vi "GenerateCode.vi"(1 "Terms":T1[](array[typedef]), 3 "Diagram":refnum<vi>, 5 "XRef":refnum<vi>, 6 "State In":T4={"Input Type"=variant(dbl 0.0), "Selection"=0, "Element Names"=[], "Type Strings"=[], "Element Types"=[]}) -> (0 "Generated Code?":bool, 2 "State Out":T4={"Input Type"=variant(dbl 0.0), "Selection"=0, "Element Names"=[], "Type Strings"=[], "Element Types"=[]}, 4 "Reply":string[](array[string]))   [LabVIEW 2015, in "Construct-Tagged-Union.xnode"]
doc: "This ability VI is called when it is time to define the execution behavior of your XNode via LabVIEW's scripting API. This VI is only called when you have previously informed LabVIEW that you need to script through a GenerateCode reply. Diagram is a reference to a diagram of a temporary VI. This diagram contains exactly one front panel terminal for each terminal of your XNode. Terms is an array of pairs of Term IDs and terminal references. LabVIEW will copy code scripted into this diagram into your XNode and connect everything to the correct terminals. The front panel terminals that are on this diagram are special in that they can only be on the top level diagram.\n \n Generate Code? is used to tell LabVIEW whether or not you want to copy the scripted diagram over. If there is an error and you wish not to commit the changes, then the old XNode behavior will be left unchanged. If you set Generate Code? to false, then this VI will be called again next time type propagation is run. Otherwise, it will not be called until you indicate that it should be through the reply on another ability VI.\n \n Because the diagram you are scripting into is separate from the VI containing the XNode instance, type propagation and the data manager will run on the temporary VI after each scripting call.\n \n You should not use the Copy scripting method to move code into the temporary VI. This will adversely affect the user's clipboard. You should use the Move scripting method instead.\n\nDefault behavior: None.\n\nThis ability does not provide UI and OS messages are not handled.\n\nSee also: ModifyCode"
uses:
  Construct-Tagged-Union.xnode
  State.ctl
  <vilib>/XNodeSupport/XNodeTermIDPair.ctl
  <vilib>/XNodeSupport/XNodeTermRef.ctl
  <vilib>/XNodeSupport/XNodeString.ctl
  <vilib>/Erdos Miller/LV-Scripting/LV-Scripting.lvlib
  <vilib>/XNodeSupport/NI_XNodeSupport.lvlib
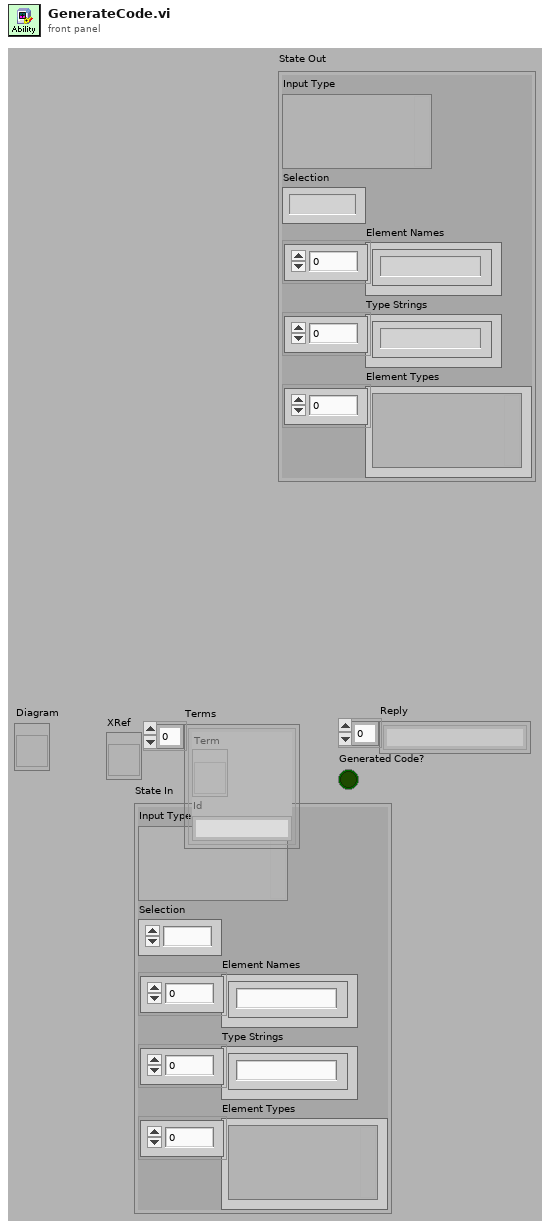
[diagram p1: front panel]
types:
  T1 = typedef "NI_XNodeSupport.lvlib/XNodeTermIDPair.ctl" = cluster{"Term":T2, "Id":T3}
  T2 = typedef "NI_XNodeSupport.lvlib/XNodeTermRef.ctl" = refnum<vi>
  T3 = typedef "NI_XNodeSupport.lvlib/XNodeString.ctl" = string
  T4 = typedef "Construct-Tagged-Union.xnode/State.ctl" = cluster{"Input Type":variant, "Selection":i32, "Element Names":string[], "Type Strings":string[], "Element Types":variant[]}
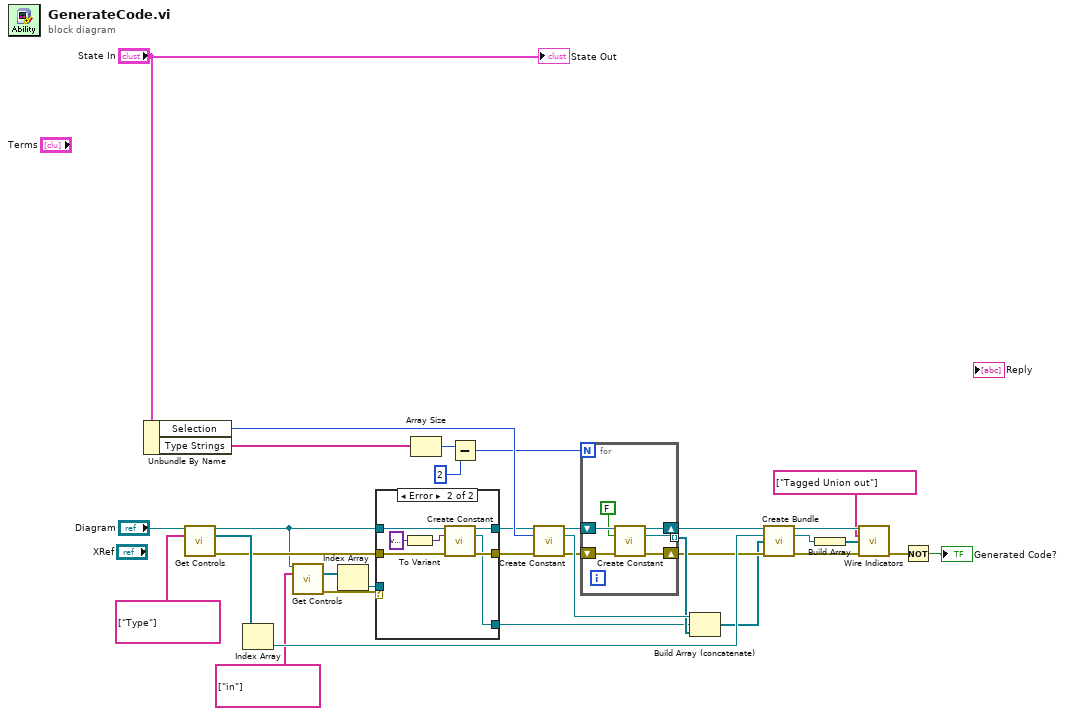
[diagram p0: block diagram]
diagram:
  n1 = Unbundle By Name("State In") -> ("Selection"=w29:i32, "Type Strings"=w27:string[])
  n2 = call <vilib>:"Get Controls.vi"("Diagram in"="Diagram", "Control Names"=string[] ["Type"]) -> ("Diagram out"=w2:refnum<vi>, "Control Terminals"=w31:refnum<vi>[], "error out"=w4:errorcluster)  [unwired: 11 in]
  n3 = Index Array(array=w31) -> (element=w20:refnum<vi>)  [unwired: 1 in]
  n4 = call <vilib>:"Get Controls.vi"("Diagram in"=w2, "Control Names"=string[] ["in"]) -> ("Control Terminals"=w8:refnum<vi>[], "error out"=w7:errorcluster)  [unwired: 11 in, 1 out]
  n5 = Index Array(array=w8) -> (element=w6:refnum<vi>)  [unwired: 1 in]
  n6 = case shown="Error" w7 {
    tunnel: [w36 w37] -> w5
    tunnel: w6 -> [w36 _]
    tunnel: w4 -> [w34 w42]
    tunnel: [w35 w40] -> w3
    tunnel: w2 -> [w35 w43]
    tunnel: [w34 w41] -> w1
    frame No Error {
    }
    frame Error {
      n7 = To Variant(anything=variant) -> (Variant=w38:variant)
      n8 = call <vilib>:"Create Constant.vi"("Diagram in"=w43, "Type"=w38, "error in (no error)"=w42) -> ("Diagram out"=w40:refnum<vi>, "Terminal"=w37:refnum<vi>, "error out"=w41:errorcluster)  [unwired: 10 in]
    }
  }
  n9 = Array Size(array=w27) -> (size(s)=w26:i32)
  n10 = Subtract(x=w26, y=2) -> (x-y=w23:i32)
  n11 = call <vilib>:"Create Constant.vi"("Diagram in"=w3, "Type"=w29, "error in (no error)"=w1) -> ("Diagram out"=w24:refnum<vi>, "Terminal"=w28:refnum<vi>, "error out"=w22:errorcluster)  [unwired: 10 in]
  n12 = for {
    N: w23 -> [_]
    shift-right: [w48] -> w19
    shift-left: w24 -> [w49]
    shift-right: [w45] -> w18
    shift-left: w22 -> [w46]
    tunnel: [w44] -> w21 mode=indexing
    n13 = call <vilib>:"Create Constant.vi"("Diagram in"=w49, "Type"=FALSE, "error in (no error)"=w46) -> ("Diagram out"=w48:refnum<vi>, "Terminal"=w44:refnum<vi>, "error out"=w45:errorcluster)  [unwired: 10 in]
  }
  n14 = Build Array (concatenate)(w28, w5, w21) -> (w17:refnum<vi>[])
  n15 = call <vilib>:"Create Bundle.vi"("Diagram in"=w19, "input cluster"=w20, "Inputs"=w17, "error in (no error)"=w18) -> ("Diagram out"=w16:refnum<vi>, "output cluster"=w11:refnum<vi>, "error out"=w15:errorcluster)  [unwired: 9 in]
  n16 = Build Array(w11) -> (w10:refnum<vi>[])
  n17 = call <vilib>:"Wire Indicators.vi"("Diagram in"=w16, "Indicator Names"=string[] ["Tagged Union out"], "Outputs"=w10, "error in (no error)"=w15) -> ("error out"=w13:errorcluster)  [unwired: 10 in, 1 out]
  n18 = Not(x=w13) -> (.not. x?=→"Generated Code?":bool)
  "State Out" <- "State In"
